vi "_Main_ByRuns_V1.1.vi"() -> ()   [LabVIEW 2017]
uses:
  <vilib>/Instr/_visa.llb/VISA Configure Serial Port (Instr).vi
panel:
  in  "WaveForm":i32(listbox)
  in  "Auto\nturn OFF":bool
  in  "6 electrodes":bool
  in  "Content":i32(listbox)
  out "LastTrigTimer, s":dbl
  in  "Graph every, cycle":dbl=10.0 min=1.0 max=100.0
  in  "SendPeriod, ms":dbl=100.0 min=10.0 max=10000.0
  out "RunsNeed":i32
  out "DAC1volt, V":dbl
  out "Time LOG":cluster{dbl[], dbl[]}(graph)
  out "LED2":bool
  out "LED1":bool
  out "TrigTimer, s":dbl
  out "Bytes at Port":u32
  out "RecTry":i32
  out "OutVoltage, V":dbl
  out "Field, kV/cm":dbl
  out "VoltageRes, V":dbl
  out "PlotPoints":cluster{"Time":dbl[], "Voltage":dbl[]}(graph)={"Time"=[0.0, 0.00037111111108161925, 0.000510833333311085, 0.0006505555555405509, 0.0007766666666915019, 0.0009172222221968695, 0.0010569444444263353, 0.0011958333333152243, 0.0013350000000274223], "Voltage"=[5.89, 5.89, 5.89, 5.89, 5.89, 5.89, 5.89, 5.89, 5.89]}
  out "VoltageBelow, V":dbl
  in  "Exposition, s":dbl=3.0
  out "Knob":u32
  out "Current, mA":dbl format="%#_4g"
  out "Channel 4, V":dbl format="%#_5g"
  out "Channel 3, V":dbl format="%#_5g"
  out "Channel 2, V":dbl format="%#_5g"
  out "Channel 1, V":dbl format="%#_5g"
  in  "Stop Button":bool
  in  "Start Button":bool
  in  "film H, nm":dbl=50.0
  out "VoltageArray, V":dbl[](array[numeric])
  out "Shutter Red":bool
  out "Shutter Green":bool
  in  "Frames In Run":u32=180
  out "Global Frame Done":u32
  out "Now is Run #":u32
  out "Frame In Run Done":u32
  in  "Step, V":dbl=1.0 min=0.01 max=50.0
  in  "Amplitude, V":dbl=1.0 min=0.1 max=50.0
  in  "LOG file":path
  in  "COM port":refnum<visa-resource-name>
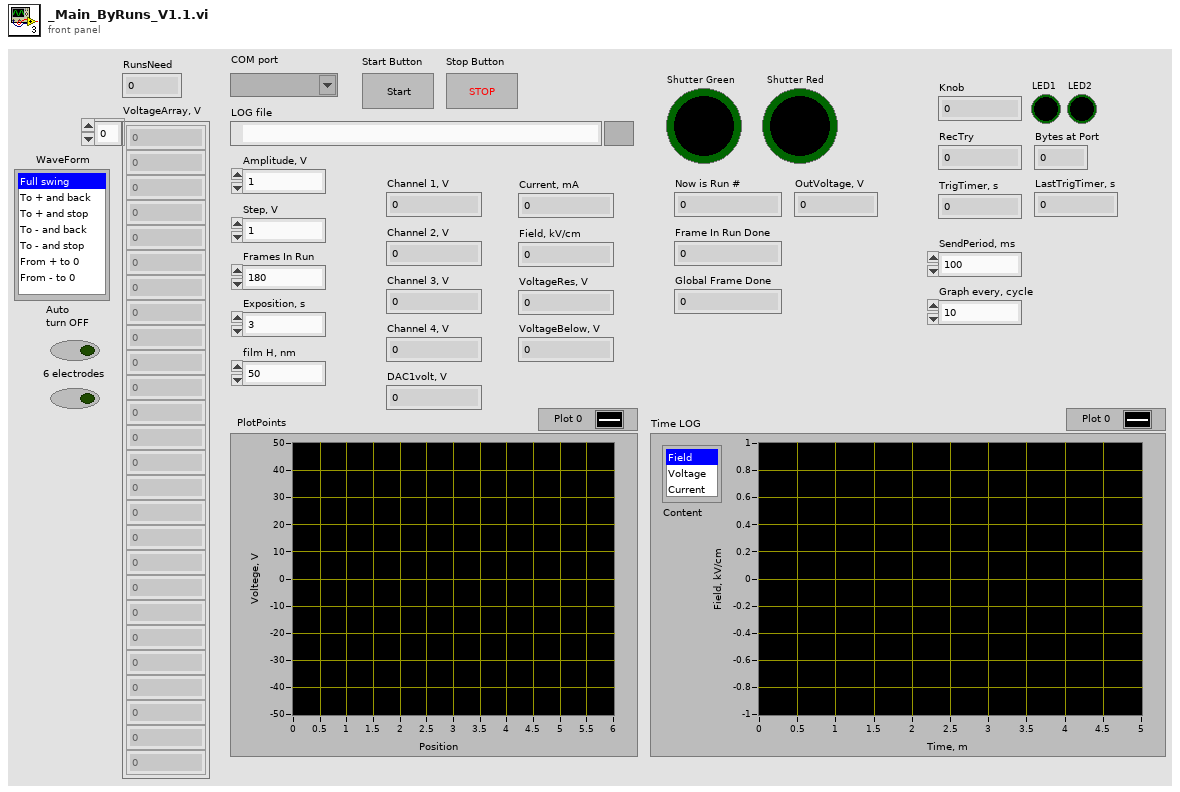
[diagram p1: front panel]
types:
  T1 = cluster{i32, i32, u32, "TrigState":bool, "TrigTimer, s":dbl, "CurrentError":bool}
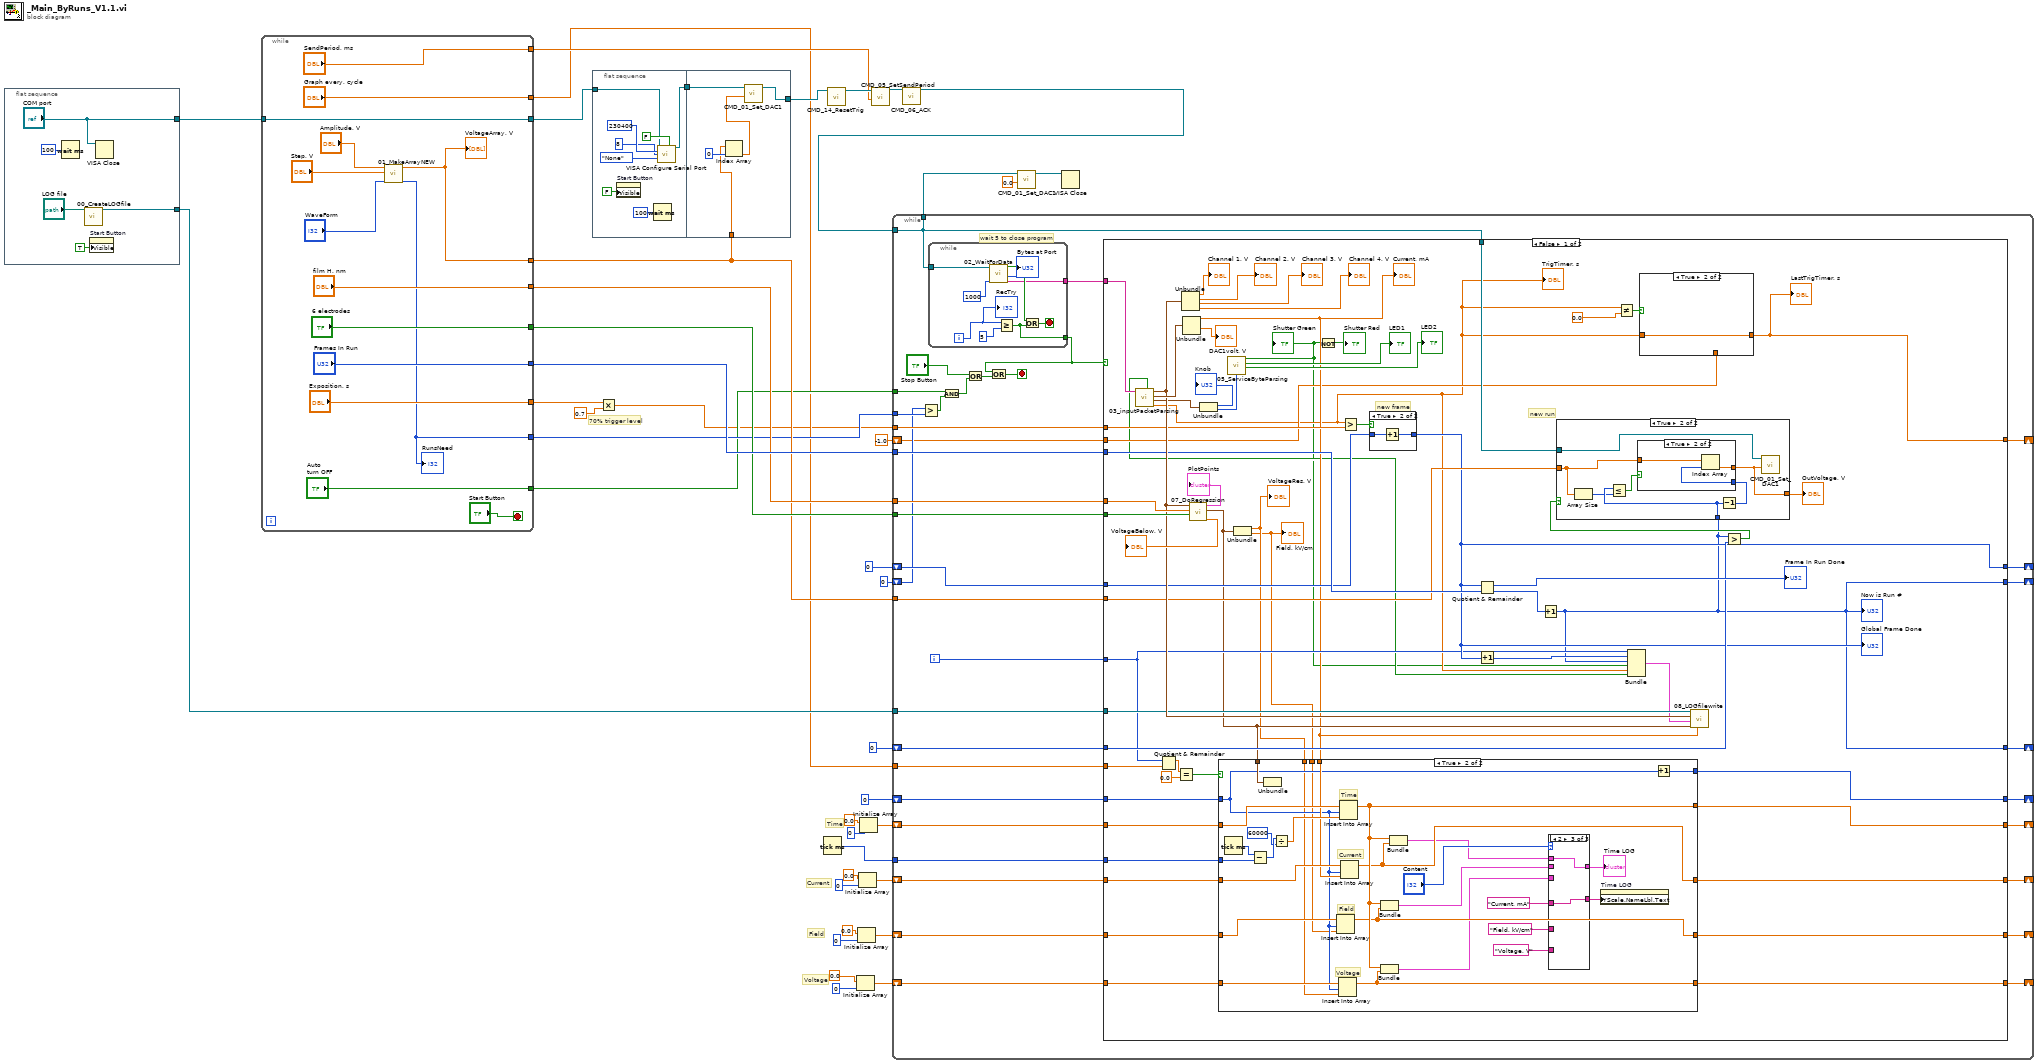
[diagram p0: block diagram]
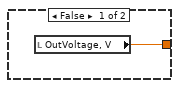
[diagram p6: hidden frame]
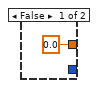
[diagram p7: hidden frame]
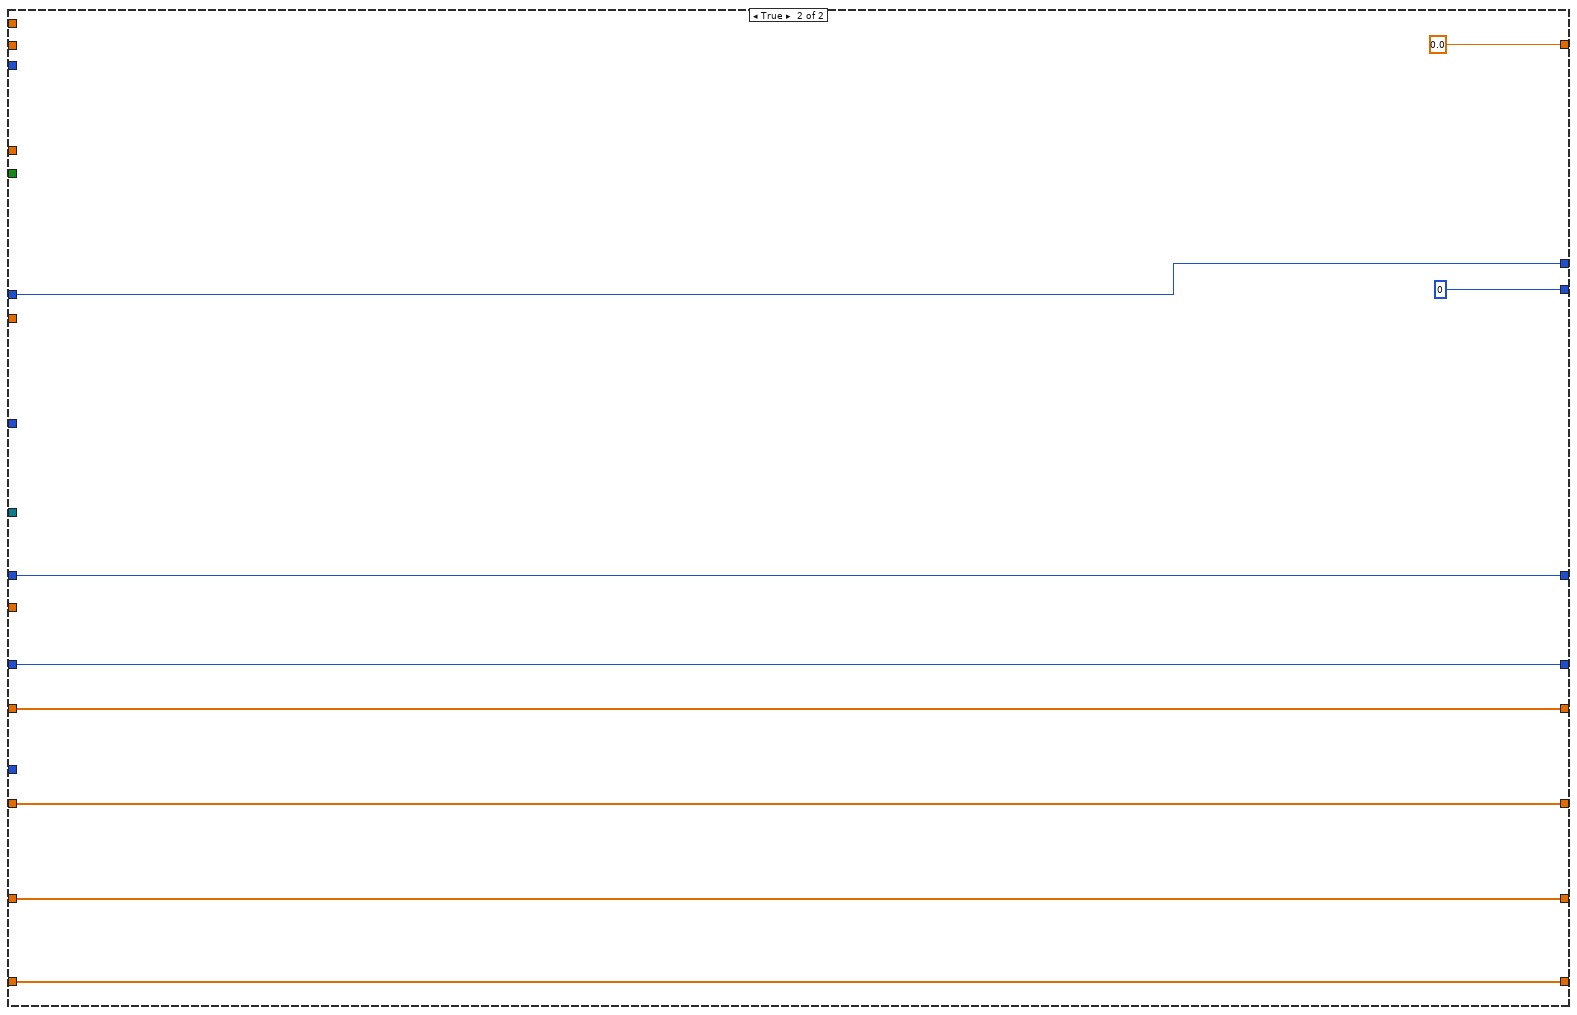
[diagram p9: hidden frame]
diagram:
  # "70% trigger level"
  # "Voltage"
  # "Field"
  # "Time"
  # "Current"
  n1 = flat-sequence {
    tunnel: ["COM port"] -> w40
    tunnel: [w42] -> w35
    frame #0 {
      n2 = Wait (ms)(milliseconds to wait=u32 100) -> ()  [unwired: 1 out]
      n3 = call "00_CreateLOGfile.vi"("LOG file"="LOG file") -> ("refnum out"=w42:refnum<file>)  [unwired: 10 in]
      n4 = property on="Start Button" class="Bool"("Visible"=TRUE) -> ()  [unwired: 2 in, 2 out]
      n5 = VISA Close(VISA resource name="COM port") -> ()  [unwired: 1 in, 1 out]
    }
  }
  n6 = while {
    tunnel: w40 -> [w50]
    tunnel: [w50] -> w39
    tunnel: [w47] -> w24
    tunnel: ["film H, nm"] -> w37
    tunnel: ["6 electrodes"] -> w36
    tunnel: ["Frames In Run"] -> w38
    tunnel: ["Exposition, s"] -> w9
    tunnel: [w46] -> w15
    tunnel: ["Auto\nturn OFF"] -> w13
    tunnel: ["SendPeriod, ms"] -> w12
    tunnel: ["Graph every, cycle"] -> w11
    stop <- "Start Button" stop-if-true
    n7 = call "01_MakeArrayNEW.vi"("Amp"="Amplitude, V", "Step"="Step, V", "WaveForm"="WaveForm") -> ("Array"=w47:dbl[], "ArraySize"=w46:i32)  [unwired: 6 in]
    "VoltageArray, V" <- w47
    "RunsNeed" <- w46
  }
  n8 = flat-sequence {
    tunnel: w39 -> [w63]
    tunnel: [w62] -> w25
    tunnel: [w70] -> w31
    tunnel: w25 -> [w69]
    tunnel: w24 -> [w68]
    frame #0 {
      n9 = property on="Start Button" class="Bool"("Visible"=FALSE) -> ()  [unwired: 2 in, 2 out]
      n10 = Wait (ms)(milliseconds to wait=u32 100) -> ()  [unwired: 1 out]
      n11 = call-poly "VISA Configure Serial Port"("VISA resource name"=w63, "Enable Termination\nChar (T)"=FALSE ("Enable Termination\nChar (T)"), "baud rate (9600)"=u32 230400, "data bits (8)"=u16 8, "parity (0:none)"=enum16{"None", "Odd", "Even", "Mark", "Space"}."None") -> ("VISA resource name out"=w62:refnum<visa-resource-name>)  [unwired: 9 in, 1 out]
    }
    frame #1 {
      n12 = Index Array(array=w68, index=0) -> (element=w72:dbl)
      n13 = call "CMD_01_Set_DAC1.vi"("Input, V"=w72, "VISA resource name"=w69) -> ("VISA resource name out"=w70:refnum<visa-resource-name>)  [unwired: 9 in]
    }
  }
  n14 = Multiply(x=w9, y=0.7) -> (x*y=w10:dbl)
  n15 = Tick Count (ms)() -> (millisecond timer value=w19:u32)
  n16 = call "CMD_14_ResetTrig.vi"("VISA resource name"=w31) -> ("VISA resource name out"=w28:refnum<visa-resource-name>)  [unwired: 10 in]
  n17 = Initialize Array(0.0 ("element"), 0 ("dimension size")) -> (w1:dbl[])
  n18 = Initialize Array(0.0 ("element"), 0 ("dimension size")) -> (w2:dbl[])
  n19 = Initialize Array(0.0 ("element"), 0 ("dimension size")) -> (w16:dbl[])
  n20 = Initialize Array(0.0 ("element"), 0 ("dimension size")) -> (w20:dbl[])
  n21 = call "CMD_05_SetSendPeriod.vi"("Period, ms"=w12, "VISA resource name"=w28) -> ("VISA resource name out"=w27:refnum<visa-resource-name>)  [unwired: 9 in]
  n22 = call "CMD_06_ACK.vi"("VISA resource name"=w27) -> ("VISA resource name out"=w26:refnum<visa-resource-name>)  [unwired: 10 in]
  n23 = while {
    tunnel: w26 -> [w95]
    tunnel: [w95] -> w32
    tunnel: w24 -> [w96]
    tunnel: w38 -> [w102]
    tunnel: w10 -> [w104]
    tunnel: w37 -> [w106]
    tunnel: w36 -> [w105]
    tunnel: w35 -> [w103]
    shift-right: [w99] -> _
    shift-left: 0 -> [w101]
    shift-right: [w98] -> _
    shift-left: u32 0 -> [w97]
    shift-right: [w93] -> _
    shift-left: 0 -> [w94]
    tunnel: w19 -> [w91]
    shift-right: [w89] -> _
    shift-left: w20 -> [w92]
    shift-right: [w88] -> _
    shift-left: w16 -> [w90]
    tunnel: w15 -> [w84]
    shift-right: [w86] -> _
    shift-left: u32 0 -> [w83]
    tunnel: w13 -> [w80]
    tunnel: w11 -> [w79]
    shift-right: [w78] -> _
    shift-left: -1.0 ("TrigTimer, s") -> [w77]
    shift-right: [w74] -> _
    shift-left: w2 -> [w76]
    shift-right: [w73] -> _
    shift-left: w1 -> [w75]
    i -> [w100]
    stop <- w109 stop-if-true
    # "wait 5 to close program"
    n24 = Greater?(x=w83, y=w84) -> (0:w81:bool)
    n25 = while {
      tunnel: w95 -> [w236]
      tunnel: [w239] -> w108
      tunnel: [w240] -> w107
      i -> [w238]
      stop <- w242 stop-if-true
      n26 = call "02_WaitForData.vi"("WaitTimeoutMS"=u32 1000, "VISA"=w236) -> ("Buffer"=w240:string, "Bytes at Port"=→"Bytes at Port":u32, "Data Recived"=w241:bool)  [unwired: 7 in]
      n27 = Greater Or Equal?(x=w238, y=5) -> (x >= y?=w239:bool)
      n28 = Or(x=w241, y=w239) -> (x .or. y?=w242:bool)
      "RecTry" <- w238
    }
    n29 = And(x=w80, y=w81) -> (x .and. y?=w82:bool)
    n30 = Or(x="Stop Button", y=w82) -> (x .or. y?=w87:bool)
    n31 = Or(x=w108, y=w87) -> (x .or. y?=w109:bool)
    n32 = case shown="False" w108 {
      tunnel: w107 -> [w170 _]
      tunnel: w106 -> [w160 _]
      tunnel: w105 -> [w159 _]
      tunnel: w104 -> [w154 _]
      tunnel: w103 -> [w157 _]
      tunnel: w102 -> [w155 _]
      tunnel: w101 -> [w152 w235]
      tunnel: w100 -> [w136 _]
      tunnel: [w143 w235] -> w99
      tunnel: [w125 w234] -> w98
      tunnel: w97 -> [w146 w234]
      tunnel: w96 -> [w148 _]
      tunnel: w95 -> [w147 _]
      tunnel: w94 -> [w134 w233]
      tunnel: [w133 w233] -> w93
      tunnel: w92 -> [w131 w232]
      tunnel: w91 -> [w130 _]
      tunnel: w90 -> [w129 w231]
      tunnel: [w127 w232] -> w89
      tunnel: [w126 w231] -> w88
      tunnel: [w125 u32 0] -> w86
      tunnel: w79 -> [w123 _]
      tunnel: [w120 0.0 ("TrigTimer, s")] -> w78
      tunnel: w77 -> [w119 _]
      tunnel: w76 -> [w115 w228]
      tunnel: w75 -> [w114 w227]
      tunnel: [w113 w228] -> w74
      tunnel: [w112 w227] -> w73
      frame False {
        # "new run"
        # "new frame"
        n33 = call "03_inputPacketParsing.vi"("string"=w170) -> ("TrigTimer, s"=w118:dbl, "Service state"=w142:cluster{u8, u8}, "DAC state"=w165:cluster{dbl, dbl, dbl, dbl}, "Voltage"=w158:cluster{dbl, dbl, dbl, dbl}, "CurrentError"=w117:bool)  [unwired: 6 in]
        "TrigTimer, s" <- w118
        n34 = Quotient & Remainder(x=w136, y=w123) -> (x-y*floor(x/y)=w138:dbl)  [unwired: 1 out]
        n35 = Equal?(x=w138, y=0.0) -> (x = y?=w135:bool)
        n36 = Unbundle(w158) -> (→"Channel 1, V":dbl, →"Channel 2, V":dbl, →"Channel 3, V":dbl, →"Channel 4, V":dbl)
        n37 = Unbundle(w165) -> (w124:dbl, →"DAC1volt, V":dbl)  [unwired: 2 out]
        "Current, mA" <- w124
        n38 = call "07_DoRegression.vi"("6 electrodes"=w159, "film H, nm"=w160, "Input ChVoltage"=w158) -> ("VoltageBelow, V"=→"VoltageBelow, V":dbl, "Regression"=w132:cluster{"VoltageRes, V":dbl, "Field, kV/cm":dbl}, "PlotPoints"=→"PlotPoints":cluster{"Time":dbl[], "Voltage":dbl[]})  [unwired: 6 in]
        n39 = Unbundle(w142) -> (→"Knob":u8, w141:u8)
        n40 = call "05_ServiceByteParsing.vi"("InputByte"=w141) -> ("LED2"=→"LED2":bool, "LED1"=→"LED1":bool, "TrigState"=w116:bool)  [unwired: 7 in, 1 out]
        "Shutter Green" <- w116
        n41 = Unbundle(w132) -> ("VoltageRes, V"=w111:dbl, "Field, kV/cm"=w110:dbl)
        "VoltageRes, V" <- w111
        "Field, kV/cm" <- w110
        n42 = case shown="True" w135 {
          tunnel: w134 -> [w177 w193]
          tunnel: [w177 w200] -> w133
          tunnel: w132 -> [_ w205]
          tunnel: w131 -> [w175 w198]
          tunnel: w130 -> [_ w203]
          tunnel: w129 -> [w176 w197]
          tunnel: [w176 w187] -> w126
          tunnel: [w175 w190] -> w127
          tunnel: w124 -> [_ w196]
          tunnel: w115 -> [w174 w195]
          tunnel: w114 -> [w173 w194]
          tunnel: [w174 w188] -> w113
          tunnel: [w173 w189] -> w112
          tunnel: w111 -> [_ w191]
          tunnel: w110 -> [_ w192]
          frame False {
          }
          frame True {
            # "Time"
            # "Voltage"
            # "Field"
            # "Current"
            n43 = Tick Count (ms)() -> (millisecond timer value=w204:u32)
            n44 = Subtract(x=w204, y=w203) -> (x-y=w202:u32)
            n45 = Unbundle(w205) -> ()  [unwired: 2 out]
            n46 = Divide(x=w202, y=u32 60000) -> (x/y=w199:dbl)
            n47 = Insert Into Array(array=w195, index=w193, new element=w192) -> (w188:dbl[])
            n48 = Insert Into Array(array=w194, index=w193, new element=w191) -> (w189:dbl[])
            n49 = Insert Into Array(array=w198, index=w193, new element=w199) -> (w190:dbl[])
            n50 = Insert Into Array(array=w197, index=w193, new element=w196) -> (w187:dbl[])
            n51 = Bundle(w190, w189) -> (w183:cluster{dbl[], dbl[]})  [unwired: 1 in]
            n52 = Bundle(w190, w188) -> (w184:cluster{dbl[], dbl[]})  [unwired: 1 in]
            n53 = Bundle(w190, w187) -> (w185:cluster{dbl[], dbl[]})  [unwired: 1 in]
            n54 = case shown="2" "Content" {
              tunnel: w185 -> [_ _ w211]
              tunnel: w184 -> [w207 _ _]
              tunnel: w183 -> [_ w209 _]
              tunnel: [w207 w209 w211] -> w182
              tunnel: "Current, mA" ("Y Scale.Name Label.Text") -> [_ _ w210]
              tunnel: "Field, kV/cm" ("Y Scale.Name Label.Text") -> [w206 _ _]
              tunnel: "Voltage, V" ("Y Scale.Name Label.Text") -> [_ w208 _]
              tunnel: [w206 w208 w210] -> w178
              frame 0, Default {
              }
              frame 1 {
              }
              frame 2 {
              }
            }
            "Time LOG" <- w182
            n55 = property on="Time LOG" class="XYGraph (strict)"("YScale.NameLbl.Text"=w178) -> ()  [unwired: 2 in, 2 out]
            n56 = Increment(x=w193) -> (x+1=w200:i32)
          }
        }
        n57 = Not(x=w116) -> (.not. x?=→"Shutter Red":bool)
        n58 = Greater?(x=w118, y=w154) -> (0:w153:bool)
        n59 = case shown="True" w153 {
          tunnel: w152 -> [w224 w226]
          tunnel: [w224 w225] -> w143
          frame False {
          }
          frame True {
            n60 = Increment(x=w226) -> (x+1=w225:i32)
          }
        }
        "Global Frame Done" <- w143
        n61 = Quotient & Remainder(x=w143, y=w155) -> (x-y*floor(x/y)=→"Frame In Run Done":u32, floor(x/y)=w150:u32)
        n62 = Increment(x=w143) -> (x+1=w144:i32)
        n63 = Increment(x=w150) -> (x+1=w125:u32)
        "Now is Run #" <- w125
        n64 = Not Equal?(x=w118, y=0.0) -> (x != y?=w122:bool)
        n65 = Bundle(w136, w144, w125, "TrigState"=w116, "TrigTimer, s"=w118, "CurrentError"=w117) -> (w156:T1)  [unwired: 1 in]
        n66 = case shown="True" w122 {
          tunnel: [w171 w172] -> w120
          tunnel: w118 -> [_ w172]
          tunnel: w119 -> [w171 _]
          frame False {
          }
          frame True {
          }
        }
        "LastTrigTimer, s" <- w120
        n67 = call "08_LOGfilewrite.vi"("DAC1cur"=w124, "Regression"=w132, "Counters"=w156, "Input ChVoltage"=w158, "refnum out"=w157) -> ()  [unwired: 7 in]
        n68 = Greater?(x=w125, y=w146) -> (0:w151:bool)
        n69 = case shown="True" w151 {
          tunnel: w148 -> [_ w215]
          tunnel: w125 -> [_ w218]
          tunnel: w147 -> [_ w214]
          tunnel: [w212 w213] -> w145
          frame False {
            n70 = local read "OutVoltage, V"() -> (w212:dbl)
          }
          frame True {
            n71 = Array Size(array=w215) -> (size(s)=w217:i32)
            n72 = Less Or Equal?(x=w218, y=w217) -> (x <= y?=w216:bool)
            n73 = Decrement(x=w218) -> (x-1=w219:u32)
            n74 = case shown="True" w216 {
              tunnel: w219 -> [_ w223]
              tunnel: w215 -> [_ w222]
              tunnel: [0.0 w221] -> w213
              frame False {
              }
              frame True {
                n75 = Index Array(array=w222, index=w223) -> (element=w221:dbl)
              }
            }
            n76 = call "CMD_01_Set_DAC1.vi"("Input, V"=w213, "VISA resource name"=w214) -> ()  [unwired: 9 in, 1 out]
          }
        }
        "OutVoltage, V" <- w145
      }
      frame True {
      }
    }
  }
  n77 = call "CMD_01_Set_DAC1.vi"("Input, V"=0.0, "VISA resource name"=w32) -> ("VISA resource name out"=w29:refnum<visa-resource-name>)  [unwired: 9 in]
  n78 = VISA Close(VISA resource name=w29) -> ()  [unwired: 1 in, 1 out]
